vi "checkResults.vi"(2 "Last Draw":i64[](array[numeric])) -> (0 "Result":i32[](array[numeric]))   [LabVIEW 2023]
uses:
  <vilib>/Utility/file.llb/Read Delimited Spreadsheet (I64).vi
panel:
  out "Your Suppose":i64[][](array[numeric])
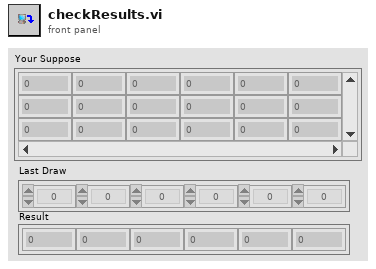
[diagram p1: front panel]
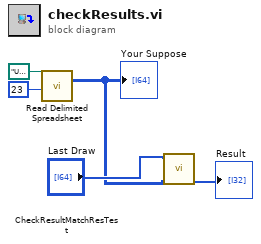
[diagram p0: block diagram]
diagram:
  n1 = call-poly <vilib>:"Read Delimited Spreadsheet.vi"("file path (dialog if empty)"=path "/Users/blagojnikolov/Desktop/@tmp/checkRes.txt", "start of read offset (chars.:0)"=23) -> ("all rows"=w2:i64[][])  [unwired: 8 in, 5 out]
  "Your Suppose" <- w2
  n2 = call "CheckResultMatchResTest.vi"("Your Suppose"=w2, "Last Draw"="Last Draw") -> ("Matches"=→"Result":i32[])  [unwired: 8 in, 1 out]
